vi "Main_Body_Wash.vi"(0 "Car_Wash_Data_In":T1) -> (4 "Car_Wash_Data_Out":T1, 6 "Do?":bool)   [LabVIEW 2023]
doc: "Updates the Main body wash process"
uses:
  Control/Car_Wash_Data.ctl
  Control/Stage_Data.ctl
  Control/Car_Wash_Indicators.ctl
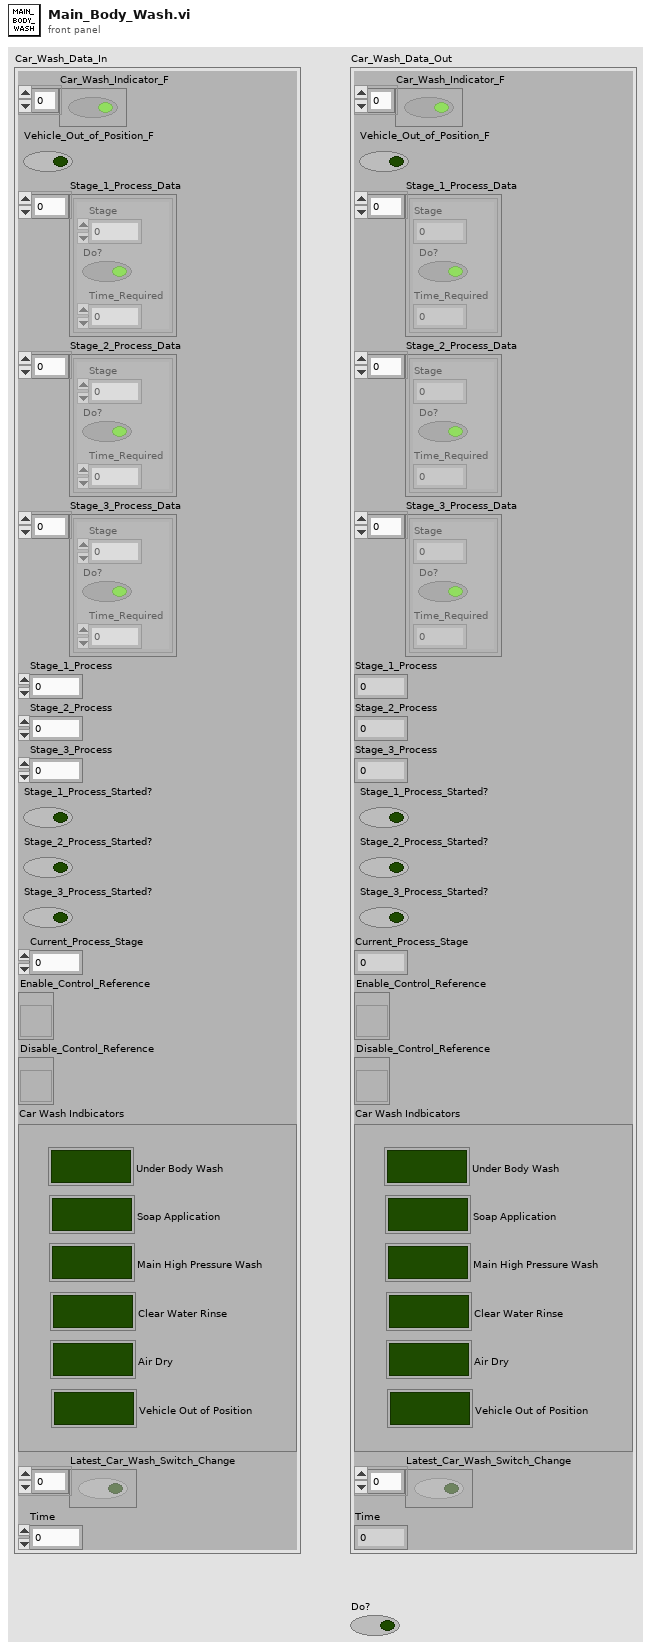
[diagram p1: front panel]
types:
  T1 = typedef "Car_Wash_Data.ctl" = cluster{"Car_Wash_Indicator_F":bool[], "Vehicle_Out_of_Position_F":bool, "Stage_1_Process_Data":T2[], "Stage_2_Process_Data":T2[], "Stage_3_Process_Data":T2[], "Stage_1_Process":i32, "Stage_2_Process":i32, "Stage_3_Process":i32, "Stage_1_Process_Started?":bool, "Stage_2_Process_Started?":bool, "Stage_3_Process_Started?":bool, "Current_Process_Stage":i32, "Enable_Control_Reference":refnum<vi>, "Disable_Control_Reference":refnum<vi>, "Car_Wash_Indicators":T3, "Latest_Car_Wash_Switch_Change":bool[], "Time":dbl}
  T2 = typedef "Stage_Data.ctl" = cluster{"Stage":i32, "Do?":bool, "Time_Required":i32}
  T3 = typedef "Car_Wash_Indicators.ctl" = cluster{"Under_Body_Wash":bool, "Soap_Application":bool, "Main_High_Pressure_Wash":bool, "Clear_Water_Rinse":bool, "Air_Dry":bool, "Vehicle_Out_of_Position":bool}
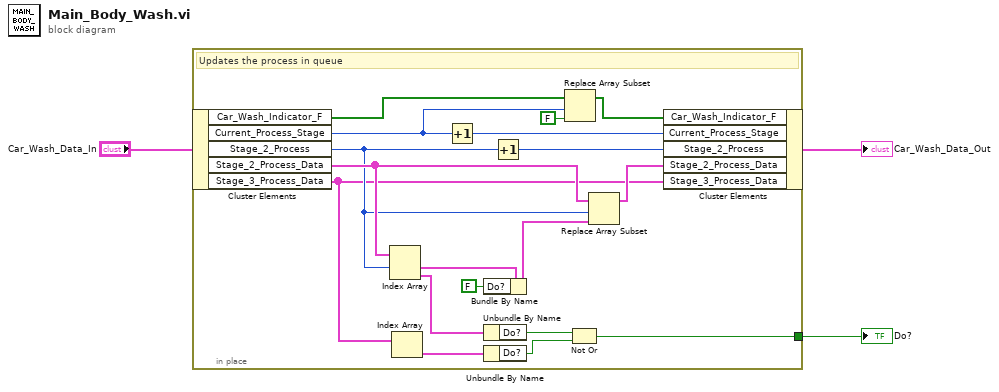
[diagram p0: block diagram]
diagram:
  n1 = in-place "In Place Element Structure" {
    in-place-border: [w8] -> w3
    # "Updates the process in queue"
    n2 = in-place-cluster #1("Car_Wash_Data_In") -> ("Car_Wash_Indicator_F"=w15:bool[], "Current_Process_Stage"=w13:i32, "Stage_2_Process"=w11:i32, "Stage_2_Process_Data"=w18:T2[], "Stage_3_Process_Data"=w5:T2[])
    n3 = Index Array(array=w18, index #1=w11) -> (element #1=w19:T2, element #2=w7:T2)  [unwired: 1 in]
    n4 = Index Array(array=w5) -> (element=w9:T2)  [unwired: 1 in]
    n5 = Increment(x=w13) -> (x+1=w21:i32)
    n6 = Bundle By Name(cluster=w19, "Do?"=FALSE) -> (w20:T2)
    n7 = Unbundle By Name(w7) -> ("Do?"=w6:bool)
    n8 = Unbundle By Name(w9) -> ("Do?"=w10:bool)
    n9 = Increment(x=w11) -> (x+1=w16:i32)
    n10 = Replace Array Subset(array=w15, new element=FALSE ("new element/subarray"), index=w13) -> (w14:bool[])
    n11 = Not Or(1:w10, 2:w6) -> (0:w8:bool)
    n12 = Replace Array Subset(array=w18, new element=w20, index=w11) -> (w17:T2[])
    n13 = in-place-cluster #1("Car_Wash_Indicator_F"=w14, "Current_Process_Stage"=w21, "Stage_2_Process"=w16, "Stage_2_Process_Data"=w17, "Stage_3_Process_Data"=w5) -> (→"Car_Wash_Data_Out":T1)
  }
  "Do?" <- w3
